vi "_ROSDefinition.vi"() -> ()   [LabVIEW 2012]
doc: "Global ROS properties"
panel:
  out "Topic History":string[](array[string])
  out "Master History":string[](array[string])
  in  "Watchdog":i32=5000
  out "Webpage Port":u16=6263
  out "Am Master?":bool
  in  "Queue Size":i32=10
  in  "TCP wait":i32=1000
  out "Servers":u16[](array[numeric])
  in  "FIFO Size":i32=10
  in  "Existing Nodes":cluster{"name":string, "Port":u16}[](array[cluster])
  out "Robot There?":bool=TRUE
  out "ROS Master":string="192.168.1.110:11311"
  # "First port is the log server"
  # "Currently disabled"
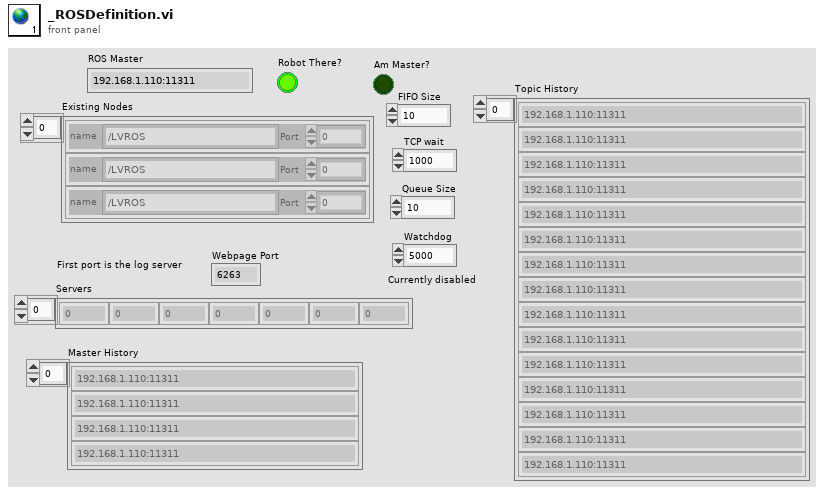
[diagram p1: front panel]
diagram:
